vi "Get2217Data.vi"(0 "CTC Node":i16=1) -> (1 "Err Msg":string, 2 "Err":bool, 3 "Ain[]":i32[](array[numeric]), 4 "Din":bool[](array[boolean]), 5 "AoutRead[]":i32[](array[numeric]), 6 "DoutRead":bool[](array[boolean]))   [LabVIEW 2011]
uses:
  Globals/SysGlbs.vi
  Globals/DCfgGlbs.vi
  Globals/DynaGlbs.vi
  Windows/System32/CTCEmcorev2.dll
panel:
  in  "clear":bool
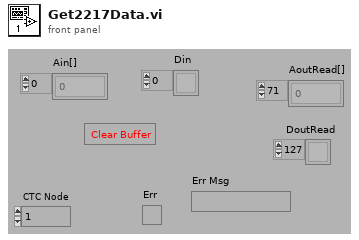
[diagram p1: front panel]
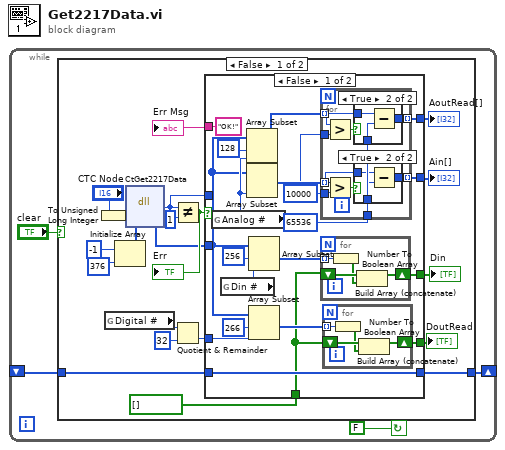
[diagram p0: block diagram]
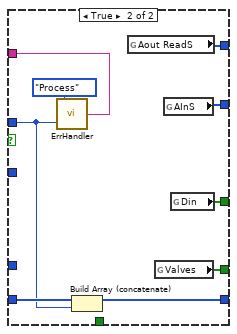
[diagram p4: hidden frame]
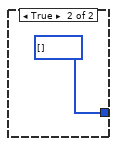
[diagram p5: hidden frame]
diagram:
  n1 = while {
    shift-left: _ -> [w3]
    shift-right: [w2] -> _
    stop <- FALSE continue-if-true
    n2 = case shown="False" "clear" {
      tunnel: w3 -> [w13 _]
      tunnel: [w12 u16[] []] -> w2
      frame False {
        n3 = To Unsigned Long Integer(number="CTC Node") -> (unsigned 32bit integer=w11:u32)
        n4 = global read "SysGlbs.vi" "Digital #"() -> (w8:u32)
        n5 = Initialize Array(-1, 376) -> (w16:i32[])
        n6 = dll-call lib="C:/Windows/System32/CTCEmcorev2.dll" fn="CtGet2217Data"("ConnectID"=w11, "Ct2217Data"=w16) -> ("return type"=w18:u32, "Ct2217Data"=w22:i32[])  [unwired: 4 in, 2 out]
        n7 = Not Equal?(x=w18, y=u32 1) -> (x != y?=w23:bool)
        "Err" <- w23
        n8 = Quotient & Remainder(x=w8, y=u32 32) -> (floor(x/y)=w6:u32)  [unwired: 1 out]
        n9 = case shown="False" w23 {
          tunnel: w22 -> [w30 _]
          tunnel: [w37 w78] -> w21
          tunnel: bool[] [] -> [w25 _]
          tunnel: [w41 w77] -> w19
          tunnel: w18 -> [_ w72]
          tunnel: ["OK!" w75] -> w17
          tunnel: w13 -> [w39 w74]
          tunnel: [w39 w73] -> w12
          tunnel: [w31 w71] -> w10
          tunnel: [w27 w70] -> w9
          tunnel: w6 -> [w26 _]
          frame False {
            w36 = 10000
            n10 = global read "SysGlbs.vi" "Analog #"() -> (w34:u32)
            n11 = global read "DCfgGlbs.vi" "Din #"() -> (w43:i32)
            n12 = Array Subset(array=w30, index=128, length=w34) -> (w32:i32[])
            n13 = Array Subset(array=w30, length=w34) -> (w38:i32[])  [unwired: 1 in]
            n14 = Array Subset(array=w30, index=256, length=w43) -> (w42:i32[])
            n15 = Array Subset(array=w30, index=266, length=w26) -> (w28:i32[])
            n16 = for {
              tunnel: w38 -> [w55] mode=indexing
              tunnel: w36 -> [w57]
              tunnel: 65536 -> [w54]
              tunnel: [w53] -> w37 mode=indexing
              tunnel: w32 -> [w52] mode=indexing
              tunnel: w36 -> [w50]
              tunnel: [w49] -> w31 mode=indexing
              n17 = Greater?(x=w52, y=w50) -> (0:w51:bool)
              n18 = Greater?(x=w55, y=w57) -> (0:w56:bool)
              n19 = case shown="True" w51 {
                tunnel: w52 -> [w58 w61]
                tunnel: w54 -> [_ w60]
                tunnel: [w58 w59] -> w49
                frame False {
                }
                frame True {
                  n20 = Subtract(x=w61, y=w60) -> (x-y=w59:i32)
                }
              }
              n21 = case shown="True" w56 {
                tunnel: w55 -> [w62 w65]
                tunnel: w54 -> [_ w64]
                tunnel: [w62 w63] -> w53
                frame False {
                }
                frame True {
                  n22 = Subtract(x=w65, y=w64) -> (x-y=w63:i32)
                }
              }
            }
            n23 = for {
              shift-right: [w67] -> w41
              shift-left: w25 -> [w68]
              tunnel: w42 -> [w69] mode=indexing
              n24 = Number To Boolean Array(number=w69) -> (Boolean array=w66:bool[])
              n25 = Build Array (concatenate)(w68, w66) -> (w67:bool[])
            }
            n26 = for {
              shift-right: [w46] -> w27
              shift-left: w25 -> [w47]
              tunnel: w28 -> [w48] mode=indexing
              n27 = Number To Boolean Array(number=w48) -> (Boolean array=w45:bool[])
              n28 = Build Array (concatenate)(w47, w45) -> (w46:bool[])
            }
          }
          frame True {
            n29 = call "ErrHandler.vi"("Err Code"=w72, "Action"=enum16{"Init", "Process"}."Process") -> ("Err Msg"=w75:string)
            n30 = Build Array (concatenate)(w74, w72) -> (w73:u32[])
            n31 = global read "DynaGlbs.vi" "Aout ReadS"() -> (w71:i32[])
            n32 = global read "DynaGlbs.vi" "Valves"() -> (w70:bool[])
            n33 = global read "DynaGlbs.vi" "AInS"() -> (w78:i32[])
            n34 = global read "DynaGlbs.vi" "Din"() -> (w77:bool[])
          }
        }
        "Ain[]" <- w21
        "Din" <- w19
        "Err Msg" <- w17
        "AoutRead[]" <- w10
        "DoutRead" <- w9
      }
      frame True {
      }
    }
  }
